vi "Transition.vi"(8 "error in (no error)":errorcluster, 9 "Target State":refnum<class "State.lvclass">, 10 "Source State":refnum<class "State.lvclass">, 11 "Local in":refnum<class "Local.lvclass">) -> (0 "error out":errorcluster, 2 "State out":refnum<class "State.lvclass">, 3 "Local out":refnum<class "Local.lvclass">)   [LabVIEW 2024, in "Transition.lvlib" / "Local.lvclass"]
uses:
  Local.lvclass
  State/State/State.lvclass
  Local.lvclass/Local.ctl
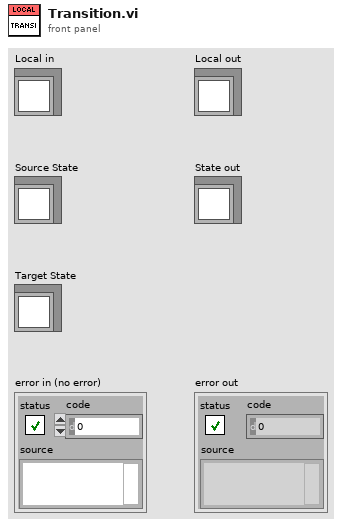
[diagram p1: front panel]
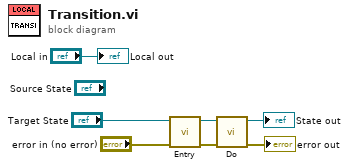
[diagram p0: block diagram]
diagram:
  n1 = call-dynamic "Entry.vi"("error in (no error)"="error in (no error)", "State in"="Target State") -> ("error out"=w2:errorcluster, "State out"=w6:refnum<class "State.lvclass">)  [unwired: 8 in]
  n2 = call-dynamic "Do.vi"("error in (no error)"=w2, "State in"=w6) -> ("error out"=→"error out":errorcluster, "State out"=→"State out":refnum<class "State.lvclass">)  [unwired: 8 in]
  "Local out" <- "Local in"
